vi "Call Function Array.vi"(8 "error in (no error)":errorcluster) -> (0 "error out":errorcluster)   [LabVIEW 2020]
uses:
  G-Embedded-Python-Interpreter-Toolkit/G-Embedded-Python-Interpreter-Toolkit.lvlib
  <vilib>/Utility/Data Type/Type Definitions/Data Type.ctl
  <vilib>/Utility/Data Type/NI_Data Type.lvlib
  G-Embedded-Python-Interpreter-Toolkit/Type Information.ctl
panel:
  out "Arguments out":cluster{u8[][][], dbl[]}
  out "Array":T1[](array[typedef])
  out "sum":u8
  out "Print Ouptut":string
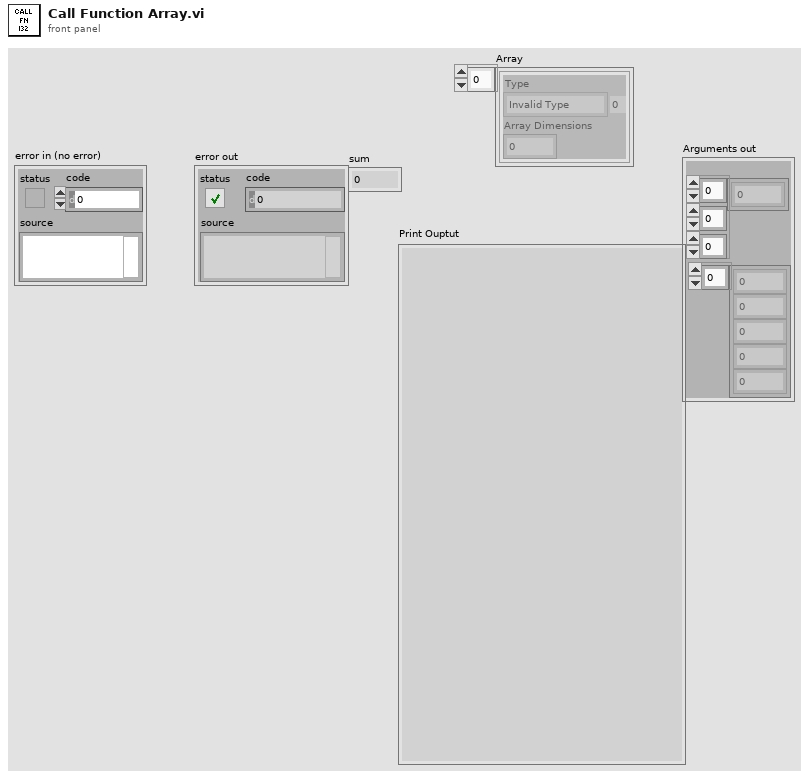
[diagram p1: front panel]
types:
  T1 = typedef "G-Embedded-Python-Interpreter-Toolkit.lvlib/Type Information.ctl" = cluster{"Type":T2, "Array Dimensions":u8}
  T2 = typedef "NI_Data Type.lvlib/Data Type.ctl" = enum8{"Invalid Type", "Void", "I8", "I16", "I32", "I64", "U8", "U16", "U32", "U64", "Single Float", "Double Float", "Extended Float", "Single Complex", "Double Complex", "Extended Complex", "Enum U8", "Enum U16", "Enum U32", "Enum U64", "Single Float With Unit", "Double Float With Unit", "Extended Float With Unit", "Single Complex with Unit", "Double Complex with Unit", "Extended Complex with Unit", "Boolean", "String", "Path", "Picture", "Tag", "Array", "Cluster", "Variant", "LV Variant", "Waveform", "Timestamp", "Digital Waveform", "Digital Data", "ExpressData", "Refnum", "External Data", "VI", "Poly VI", "LabVIEW Class Instance", "Fixed Point", "Set Collection", "Map Collection"}
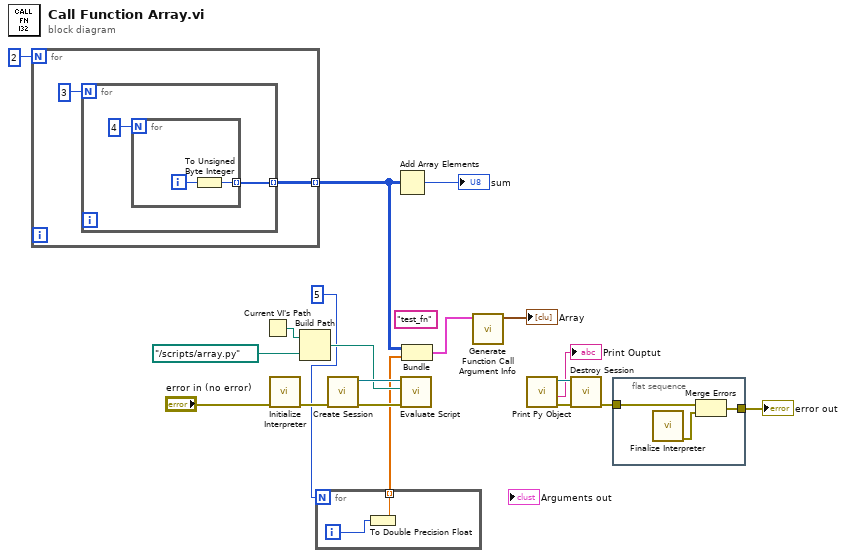
[diagram p0: block diagram]
diagram:
  (unwired) "test_fn" ("Label")
  n1 = for {
    N: 2 -> [_]
    tunnel: [w21] -> w6 mode=indexing
    n2 = for {
      N: 3 -> [_]
      tunnel: [w23] -> w21 mode=indexing
      n3 = for {
        N: 4 -> [_]
        tunnel: [w24] -> w23 mode=indexing
        i -> [w25]
        n4 = To Unsigned Byte Integer(number=w25) -> (unsigned 8bit integer=w24:u8)
      }
    }
  }
  n5 = Current VI's Path() -> (path=w16:path)
  n6 = call "Initialize Interpreter.vi"("error in (no error)"="error in (no error)") -> ("error out"=w18:errorcluster)  [unwired: 9 in, 1 out]
  n7 = Build Path(base path=w16, name or relative path=path "../scripts/array.py" ("Path")) -> (appended path=w14:path)
  n8 = for {
    N: 5 ("dimension size") -> [_]
    tunnel: [w26] -> w1 mode=indexing
    i -> [w27]
    n9 = To Double Precision Float(number=w27) -> (double precision float=w26:dbl)
  }
  n10 = call "Create Session.vi"("error in (no error)"=w18) -> ("error out"=w13:errorcluster, "Session Handle"=w17:refnum<data-value>)  [unwired: 9 in]
  n11 = Add Array Elements(numeric array=w6) -> (sum=→"sum":u8)
  n12 = call "Evaluate Script.vi"("error in (no error)"=w13, "Script File Path"=w14, "Session Handle in"=w17) -> ()  [unwired: 7 in, 2 out]
  n13 = Bundle(w6, w1) -> (w5:cluster{u8[][][], dbl[]})  [unwired: 1 in]
  n14 = call "Generate Function Call Argument Info.vi"("Data Type"=w5) -> ("Array"=→"Array":T1[])  [unwired: 9 in, 1 out]
  n15 = call "Print Py Object.vi"() -> ("error out"=w9:errorcluster, "Print Ouptut"=→"Print Ouptut":string, "Session Handle out"=w10:refnum<data-value>)  [unwired: 8 in, 1 out]
  n16 = call "Destroy Session.vi"("error in (no error)"=w9, "Session Handle"=w10) -> ("error out"=w12:errorcluster)  [unwired: 9 in]
  n17 = flat-sequence {
    tunnel: w12 -> [w30]
    tunnel: [w28] -> w19
    frame #0 {
      n18 = call "Finalize Interpreter.vi"() -> ("error out"=w29:errorcluster)  [unwired: 11 in]
      n19 = Merge Errors(w30, w29) -> (w28:errorcluster)
    }
  }
  "error out" <- w19
